vi "ServerCreateProcess.vi"(7 "Process Header":string, 9 "error in (no error)":errorcluster) -> (0 "Process Reference":refnum<vi>, 2 "Process Name":string, 6 "error out":errorcluster)   [LabVIEW 2009]
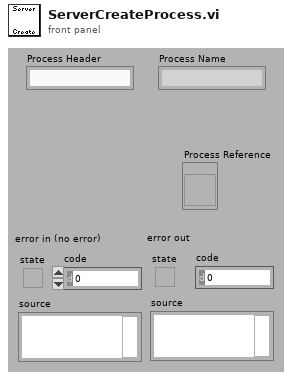
[diagram p1: front panel]
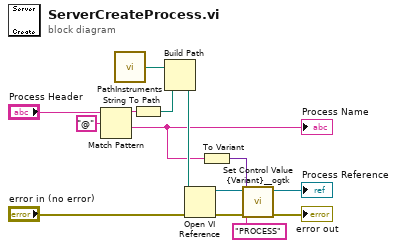
[diagram p0: block diagram]
diagram:
  n1 = Match Pattern(string="Process Header", regular expression="@" ("expression régulière")) -> (before substring=w13:string, after substring=w4:string)  [unwired: 3 out]
  "Process Name" <- w4
  n2 = call "PathInstruments.vi"() -> ("Instruments Path"=w3:path)
  n3 = String To Path(string=w13) -> (path=w9:path)
  n4 = Build Path(base path=w3, name or relative path=w9) -> (appended path=w10:path)
  n5 = Open VI Reference(vi path=w10, error in (no error)="error in (no error)") -> (vi reference=w6:refnum<vi>, error out=w7:errorcluster)  [unwired: 4 out]
  n6 = To Variant(anything=w4) -> (Variant=w5:variant)
  n7 = call <userlib>:"Set Control Value {Variant}__ogtk.vi"("error in (no error)"=w7, "Control Name (\"\": use variant name)"="PROCESS" ("Control Name"), "Value"=w5, "VI Refnum"=w6) -> ("error out"=→"error out":errorcluster, "VI Refnum dup"=→"Process Reference":refnum<vi>)  [unwired: 6 out]
